vi "Execute.vi"(8 "error in (no error)":errorcluster, 9 "Consumer Queues in":T1, 10 "DAC Process Command in":refnum<class "Configure DAC Test Stand.lvclass">, 11 "DAC Process Data in":T2) -> (0 "error out":errorcluster, 1 "Consumer Queues out":T1, 2 "Stop?":bool, 3 "DAC Process Data out":T2)   [LabVIEW 2019, in "DAC Process.lvlib" / "Configure DAC Test Stand.lvclass"]
uses:
  Configure DAC Test Stand.lvclass
  Generic DAC Command/Generic DAC Process Command.lvclass
  Generic Test Stand/Generic Test Stand.lvclass
  Trig Process/Config and Run TRIG Process/Config and Run TRIG Process.lvclass
  Trig Process/Stop TRIG/Stop TRIG.lvclass
  DAC Process Data.ctl
  DAC Process.lvlib
  UI Process/Generic UI Command/Generic UI Process Command.lvclass
  TS Framework/Consumer Queues.ctl
  TS Framework/TS Framework.lvlib
  TS Framework/ExeLogging/DAC Logger/DAC Logger.lvclass
  DAC State.ctl
  Trig Process/Generic Trig Command/Generic Trig Process Command.lvclass
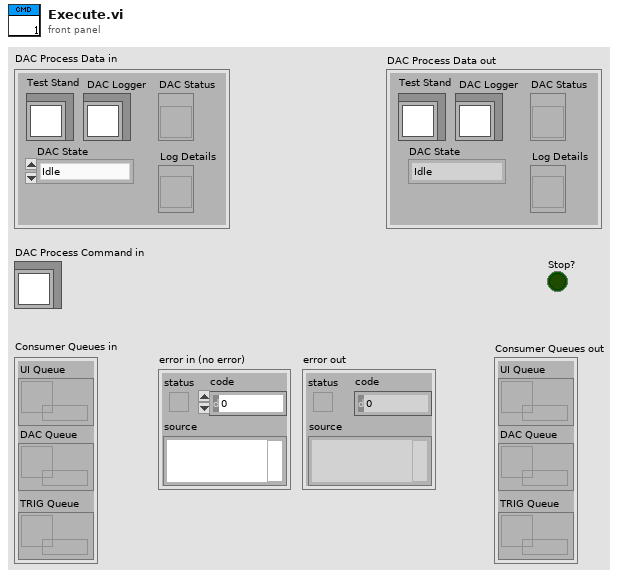
[diagram p1: front panel]
types:
  T1 = typedef "TS Framework.lvlib/Consumer Queues.ctl" = cluster{"UI Queue":refnum<queue>, "DAC Queue":refnum<queue>, "TRIG Queue":refnum<queue>}
  T2 = typedef "DAC Process.lvlib/DAC Process Data.ctl" = cluster{"Test Stand":refnum<class "Generic Test Stand.lvclass">, " DAC Logger":refnum<class "DAC Logger.lvclass">, "DAC State":T3, "DAC Status":refnum<vi>, "Log Details":refnum<vi>}
  T3 = typedef "DAC Process.lvlib/DAC State.ctl" = enum16{"Idle", "Acquiring"}
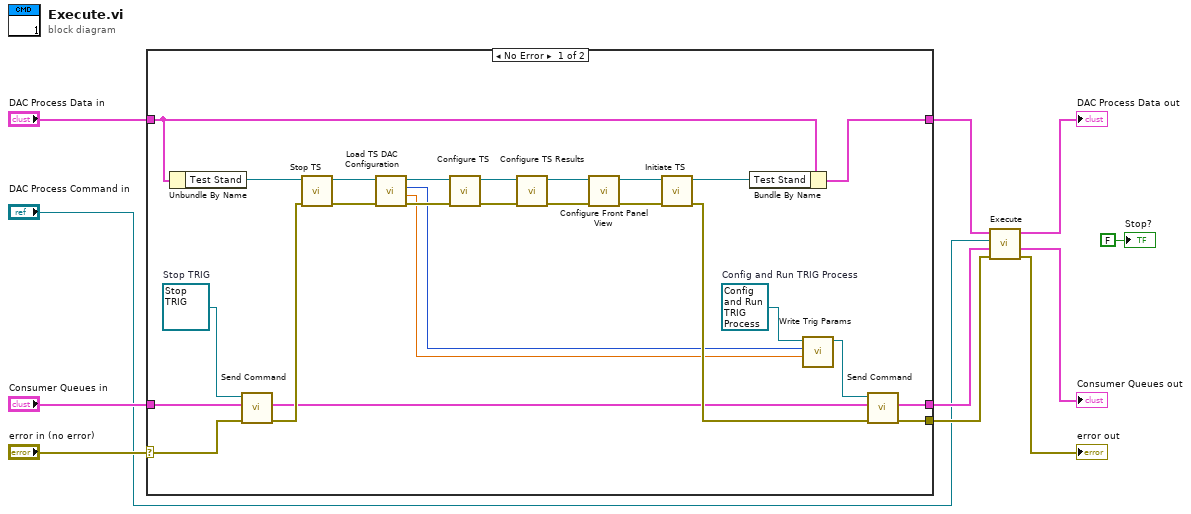
[diagram p0: block diagram]
diagram:
  n1 = case shown="No Error" "error in (no error)" {
    selector: "error in (no error)" -> [w16 w40]
    tunnel: [w27 w40] -> w6
    tunnel: "Consumer Queues in" -> [w18 w39]
    tunnel: [w29 w39] -> w5
    tunnel: "DAC Process Data in" -> [w32 w38]
    tunnel: [w30 w38] -> w3
    frame No Error {
      w17 = refnum<class "Stop TRIG.lvclass"> refnum  # Stop TRIG
      w26 = refnum<class "Config and Run TRIG Process.lvclass"> refnum  # Config and Run TRIG Process
      n2 = Unbundle By Name(w32) -> ("Test Stand"=w34:refnum<class "Generic Test Stand.lvclass">)
      n3 = call-dynamic "Send Command.vi"("error in (no error)"=w16, "Consumer Queues in"=w18, "Trig Process Command"=w17) -> ("error out"=w15:errorcluster, "Consumer Queues out"=w14:T1)  [unwired: 7 in]
      n4 = call-dynamic "Stop TS.vi"("error in (no error)"=w15, "Generic Test Stand in"=w34) -> ("error out"=w35:errorcluster, "Generic Test Stand out"=w33:refnum<class "Generic Test Stand.lvclass">)  [unwired: 8 in]
      n5 = call-dynamic "Load TS DAC Configuration.vi"("error in"=w35, "Test Stand in"=w33) -> ("error out"=w36:errorcluster, "Ctrl Interval"=w12:dbl, "Trig Resolution"=w13:u32, "Test Stand out"=w37:refnum<class "Generic Test Stand.lvclass">)  [unwired: 6 in]
      n6 = call-dynamic "Configure TS.vi"("error in"=w36, "Test Stand in"=w37) -> ("error out"=w21:errorcluster, "Test Stand out"=w22:refnum<class "Generic Test Stand.lvclass">)  [unwired: 8 in]
      n7 = call-dynamic "Configure TS Results.vi"("error in"=w21, "Test Stand in"=w22) -> ("error out"=w19:errorcluster, "Test Stand out"=w20:refnum<class "Generic Test Stand.lvclass">)  [unwired: 8 in]
      n8 = call-dynamic "Configure Front Panel View.vi"("error in"=w19, "Generic Test Stand in"=w20) -> ("error out"=w23:errorcluster, "Generic Test Stand out"=w24:refnum<class "Generic Test Stand.lvclass">)  [unwired: 8 in]
      n9 = call-dynamic "Initiate TS.vi"("error in (no error)"=w23, "Generic Test Stand in"=w24) -> ("error out"=w28:errorcluster, "Generic Test Stand out"=w31:refnum<class "Generic Test Stand.lvclass">)  [unwired: 8 in]
      n10 = Bundle By Name(cluster=w32, "Test Stand"=w31) -> (w30:T2)
      n11 = call "Write Trig Params.vi"("Ctrl Interval"=w12, "Trig Resolution"=w13, "Config and Run TRIG Process in"=w26) -> ("Config and Run TRIG Process out"=w25:refnum<class "Config and Run TRIG Process.lvclass">)  [unwired: 7 in, 1 out]
      n12 = call-dynamic "Send Command.vi"("error in (no error)"=w28, "Consumer Queues in"=w14, "Trig Process Command"=w25) -> ("error out"=w27:errorcluster, "Consumer Queues out"=w29:T1)  [unwired: 7 in]
    }
    frame Error {
    }
  }
  n13 = call-parent "Execute.vi"("error in"=w6, "Consumer Queues in"=w5, "DAC Process Command in"="DAC Process Command in", "DAC Process Data in"=w3) -> ("error out"=→"error out":errorcluster, "Consumer Queues out"=→"Consumer Queues out":T1, "DAC Process Data out"=→"DAC Process Data out":T2)  [unwired: 4 in, 1 out]
  "Stop?" <- FALSE ("Stop?")
